vi "WavefromProps.vi"(11 "signal in":waveform(dbl)) -> (2 "Waveform Properties":T1, 3 "signal out":waveform(dbl))   [LabVIEW 2014, in "XListGraph.lvlib" / "XListGraph.xctl"]
uses:
  XListGraph.xctl
  def-wfProps.ctl
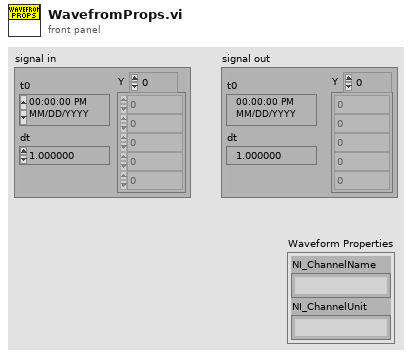
[diagram p1: front panel]
types:
  T1 = typedef "XListGraph.lvlib/XListGraph.xctl/def-wfProps.ctl" = cluster{"NI_ChannelName":string, "NI_ChannelUnit":string}
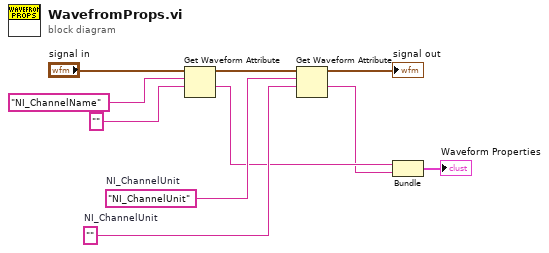
[diagram p0: block diagram]
diagram:
  w5 = "NI_ChannelUnit"  # NI_ChannelUnit
  w4 = ""  # NI_ChannelUnit
  n1 = Get Waveform Attribute(5:"", 6:"NI_ChannelName", 7:"signal in") -> (1:w2:string, 3:w7:waveform(dbl))  [unwired: 1 in, 2 out]
  n2 = Get Waveform Attribute(5:w4, 6:w5, 7:w7) -> (1:w1:string, 3:→"signal out":waveform(dbl))  [unwired: 1 in, 2 out]
  n3 = Bundle(w2, "NI_ChannelUnit"=w1) -> (→"Waveform Properties":cluster{string, "NI_ChannelUnit":string})  [unwired: 1 in]
